vi "gentec-SOLO-PE.Scaler.vi"(1 "Scaler":u32, 2 "Value":u32) -> (0 "Scaled Value":dbl format="%.12f")   [LabVIEW 2014, in "gentec-SOLO-PE - Driver.lvlib"]
uses:
  gentec-SOLO-PE - Driver.lvlib
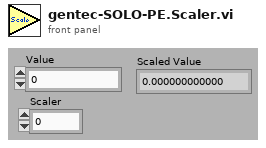
[diagram p1: front panel]
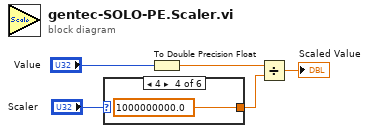
[diagram p0: block diagram]
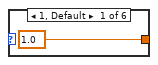
[diagram p2: hidden frame]
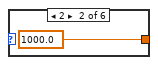
[diagram p3: hidden frame]
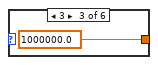
[diagram p4: hidden frame]
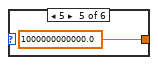
[diagram p5: hidden frame]
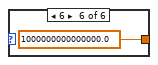
[diagram p6: hidden frame]
diagram:
  n1 = case shown="4" "Scaler" {
    tunnel: [1.0 1000.0 1000000.0 1000000000.0 1000000000000.0 1000000000000000.0] -> w2
    frame 1, Default {
      (unwired) " "
    }
    frame 2 {
    }
    frame 3 {
    }
    frame 4 {
    }
    frame 5 {
    }
    frame 6 {
    }
  }
  n2 = To Double Precision Float(number="Value") -> (double precision float=w3:dbl)
  n3 = Divide(x=w3, y=w2) -> (x/y=→"Scaled Value":dbl)
